vi "Write_XY_Max.vi"(6 "Numeric 2":dbl, 7 "Numeric":dbl, 9 "Integer Time":i64, 10 "X-Y position":dbl[](array[numeric]), 11 "XY and Max":path=path "C:/Users/Chris/Desktop/DCS(Upgrade)/dcs_points/dcs_points.csv") -> ()   [LabVIEW 2013]
uses:
  <vilib>/Utility/file.llb/Write To Spreadsheet File (DBL).vi
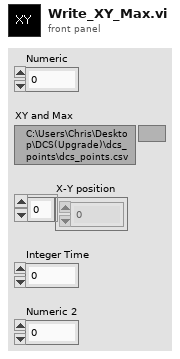
[diagram p1: front panel]
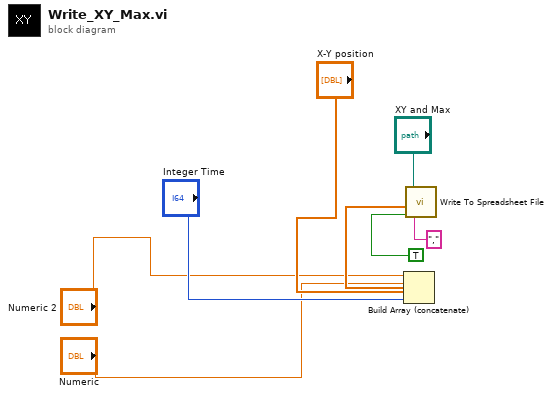
[diagram p0: block diagram]
diagram:
  n1 = Build Array (concatenate)("Numeric 2", "Numeric", "X-Y position", "Integer Time") -> (w3:dbl[])
  n2 = call-poly <vilib>:"Write To Spreadsheet File.vi"("delimiter (\\t)"="," ("delimiter (\\t)"), "append to file? (new file:F)"=TRUE, "1D data"=w3, "file path (dialog if empty)"="XY and Max") -> ()  [unwired: 4 in, 1 out]
